vi "Add Projectname.vi"() -> ()   [LabVIEW 2011]
panel:
  in  "path":path
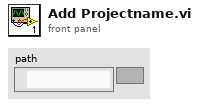
[diagram p1: front panel]
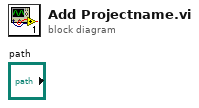
[diagram p0: block diagram]
diagram:
